vi "Sequencer.vi"() -> ()   [LabVIEW 2019]
uses:
  Sequencer mode.ctl
  Axis driver/Xeryon Axis command.ctl
  Serial driver/Xeryon serial command.ctl
panel:
  in  "Exit":bool
  out "Within tolerance":bool
  in  "Stop":bool
  in  "Apply default file":bool
  in  "Settings default":path
  out "Position reached":bool
  in  "Stage selector":string
  out "Current pos":dbl
  in  "# cycles":u16
  out "Cycle":u16
  in  "Speed":dbl
  in  "Position 2":dbl
  in  "Position 1":dbl
  in  "Start":bool
  in  "Current status":T1
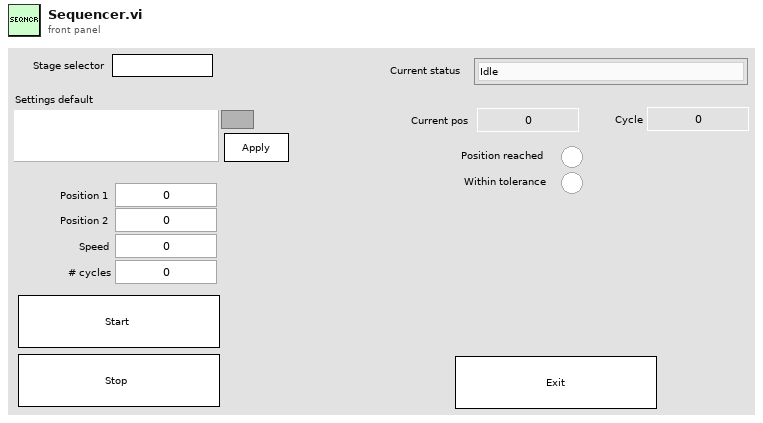
[diagram p1: front panel]
types:
  T1 = typedef "Sequencer mode.ctl" = enum16{"Idle", "-", "Go to first pos", "Moving to first position", "Go to 2nd pos", "Moving to 2nd position", "Check what's next"}
  T2 = typedef "Xeryon Axis command.ctl" = cluster{"Command":enum16{"Reset", "Zero output", "Go home", "Find index", "Scan -X", "Scan +X", "Scan Stop", "Step -X", "Step +X", "Set DPOS", "Stop", "Continue", "Desired speed", "Apply settings file", "Exit", "Reset encoder", "Recover", "Save"}, "Data to send":string}
  T3 = typedef "Xeryon serial command.ctl" = cluster{"Command":enum16{"Send serial data", "Exit"}, "Data to send":string}
  T4 = enum16{"Init", "Set stage data", "Update position", "Get"}
  T5 = typedef "Xeryon status bits.ctl" = cluster{"Amplifiers enabled":bool, "End stop":bool, "Thermal protection 1":bool, "Thermal protection 2":bool, "Force zero":bool, "Motor On":bool, "Closed loop":bool, "Encoder at index":bool, "Encoder valid":bool, "Searching index":bool, "Position reached":bool, "Error compensation":bool, "Encoder error":bool, "Scanning":bool, "Left end stop":bool, "Right and stop":bool, "Error limit":bool, "Searching optimal frequency":bool, "Safety timeout triggered":bool, "EtherCAT acknowledge":bool, "Emergency stop":bool, "Position fail":bool}
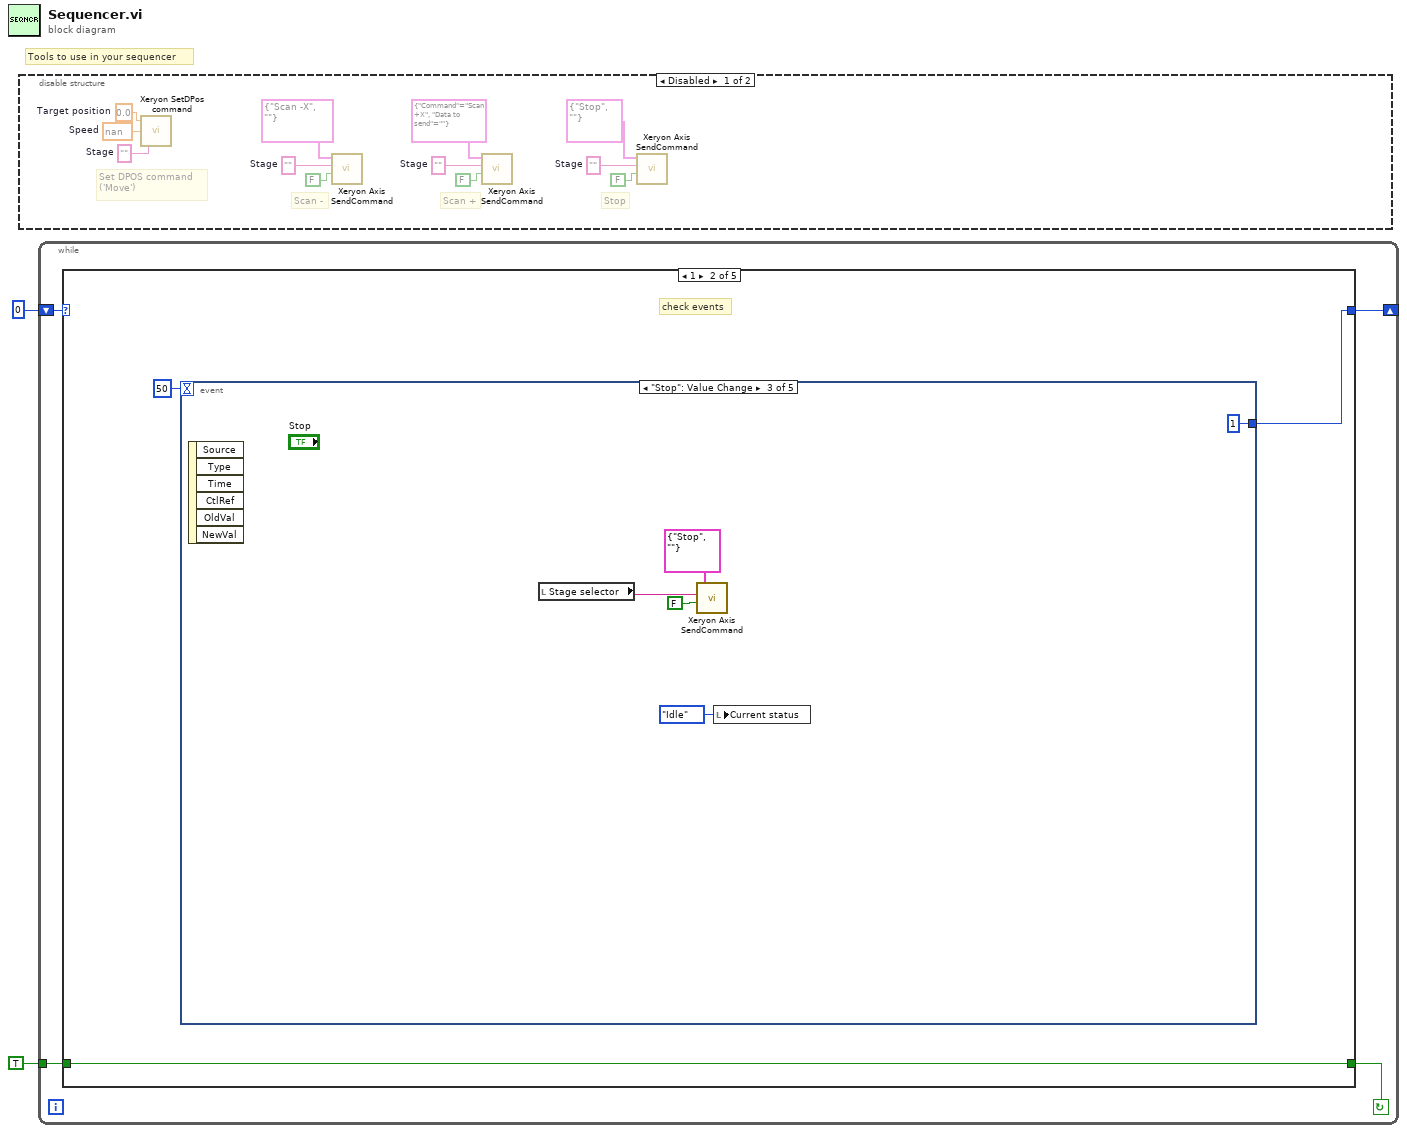
[diagram p0: block diagram]
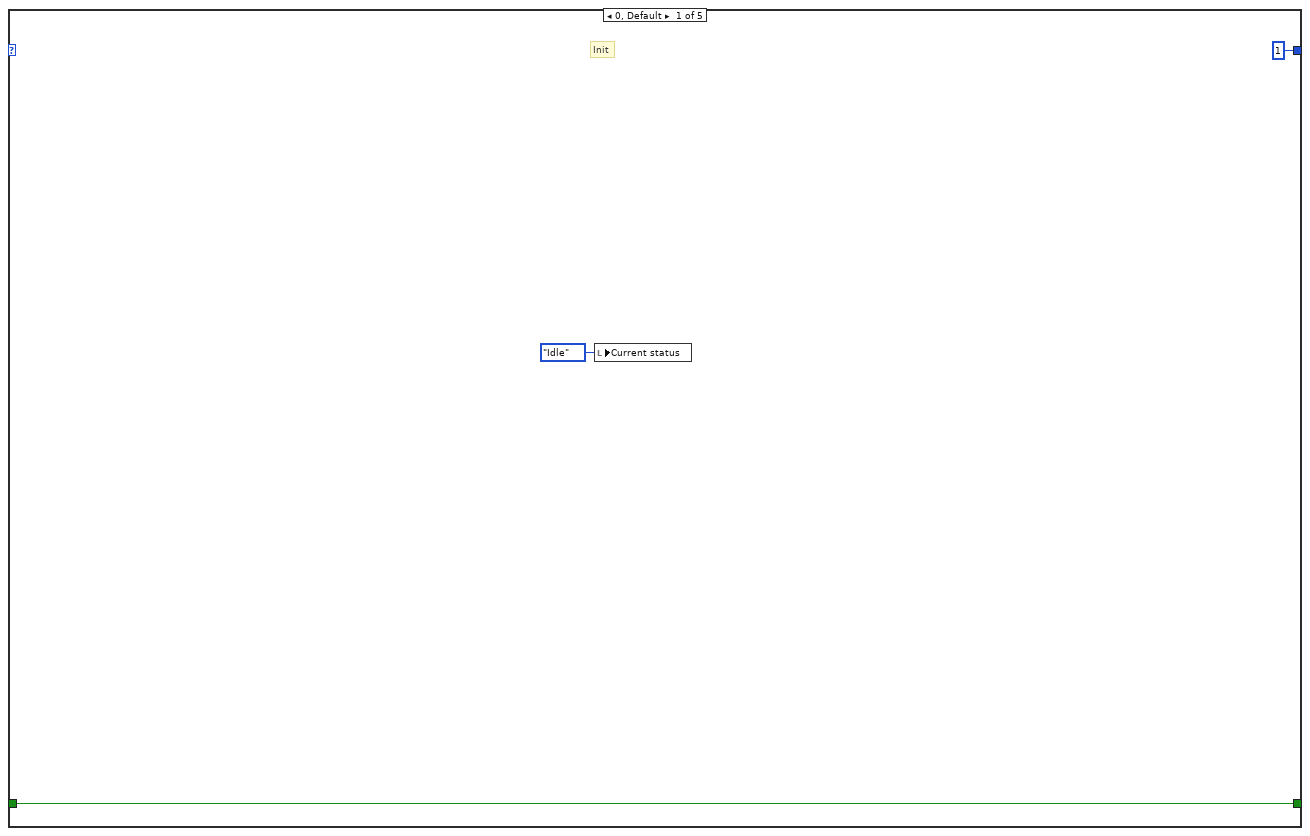
[diagram p3: hidden frame]
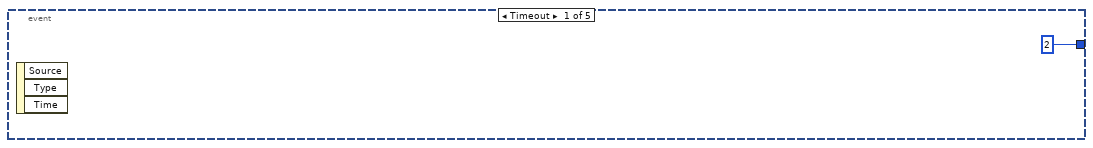
[diagram p4: hidden frame]
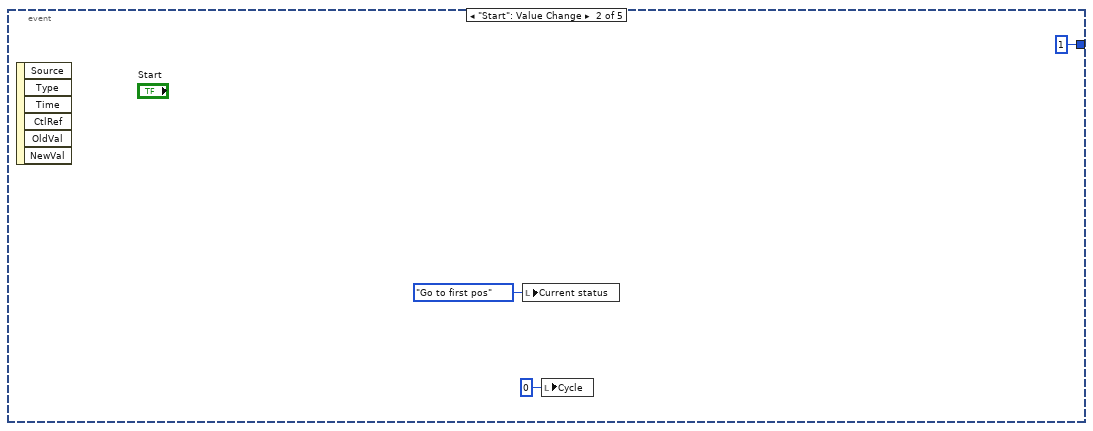
[diagram p5: hidden frame]
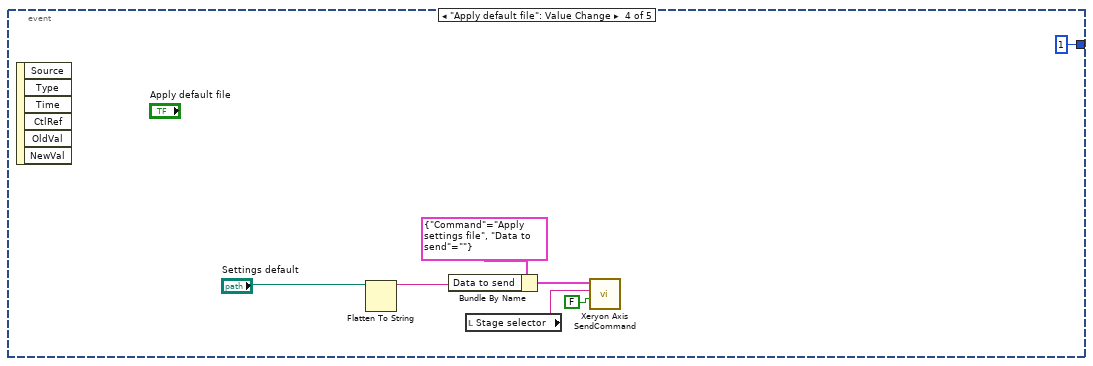
[diagram p6: hidden frame]
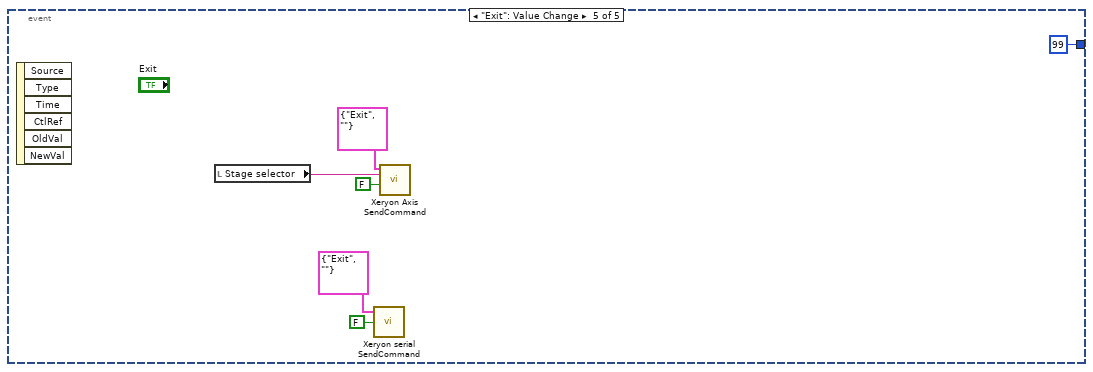
[diagram p7: hidden frame]
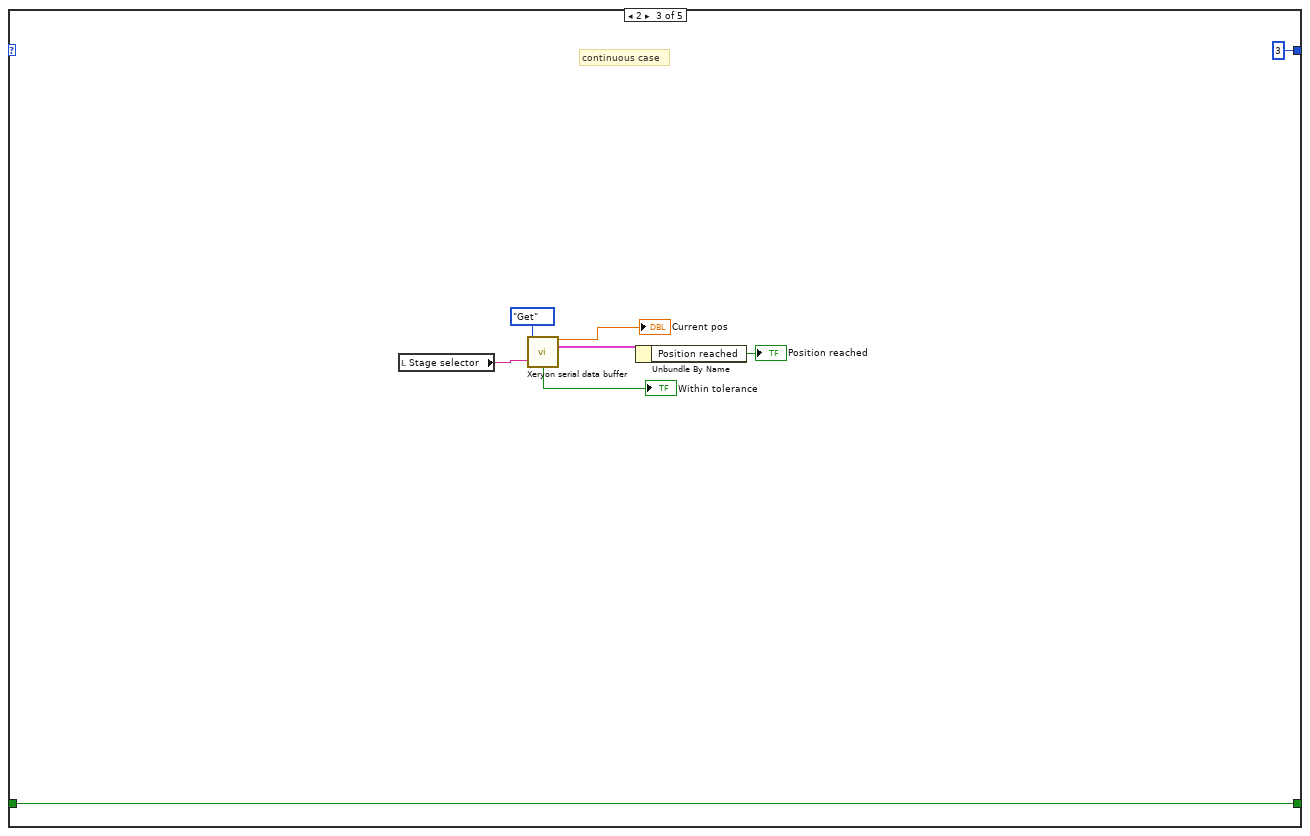
[diagram p8: hidden frame]
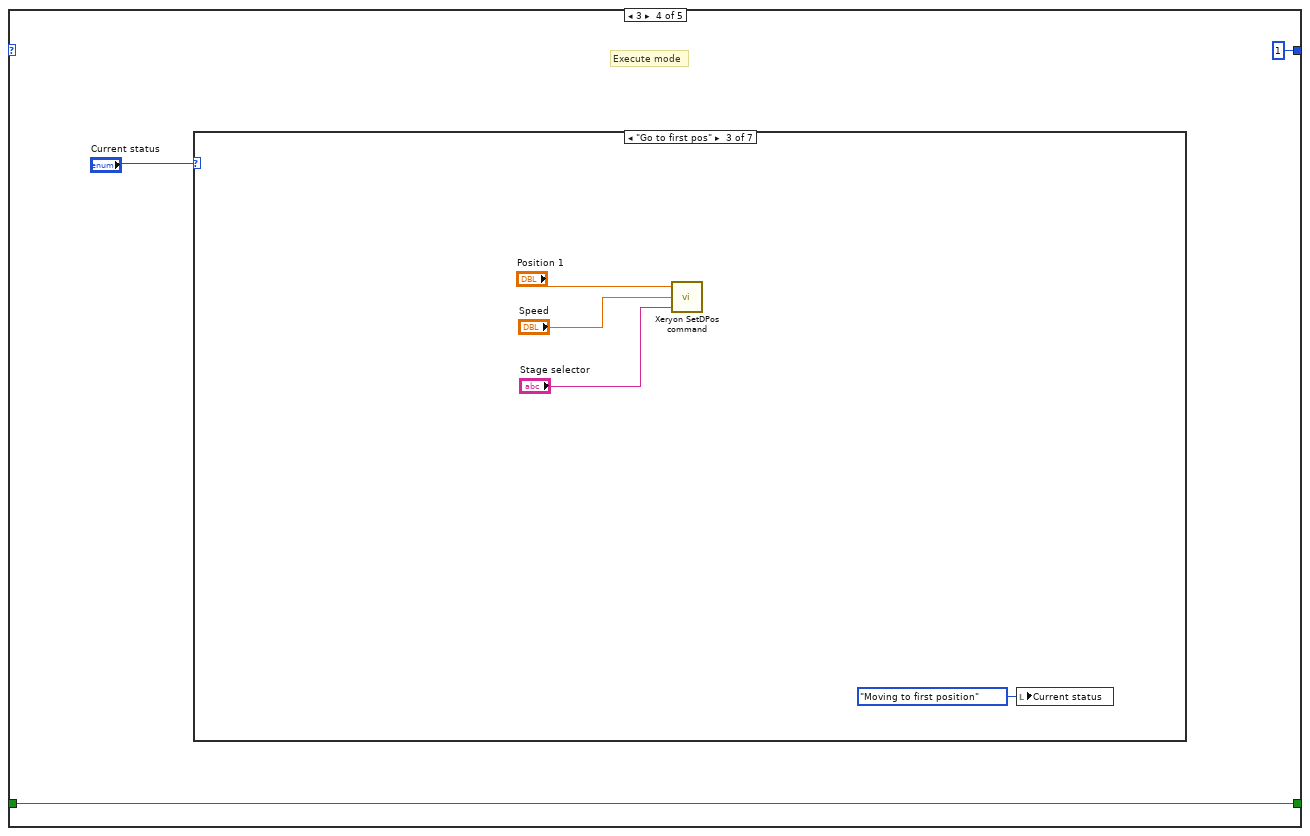
[diagram p9: hidden frame]
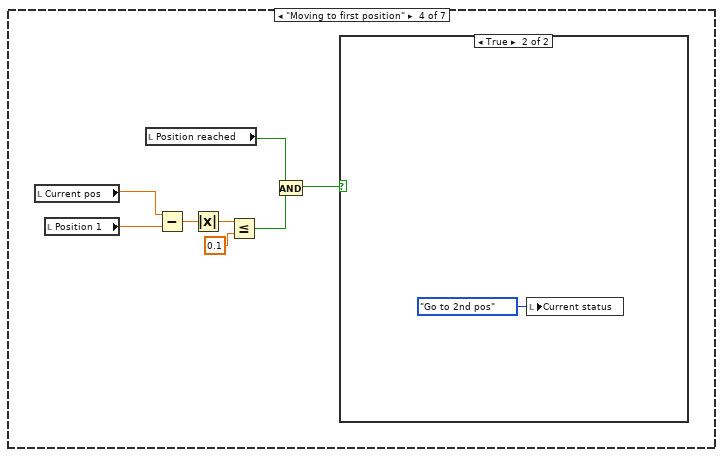
[diagram p12: hidden frame]
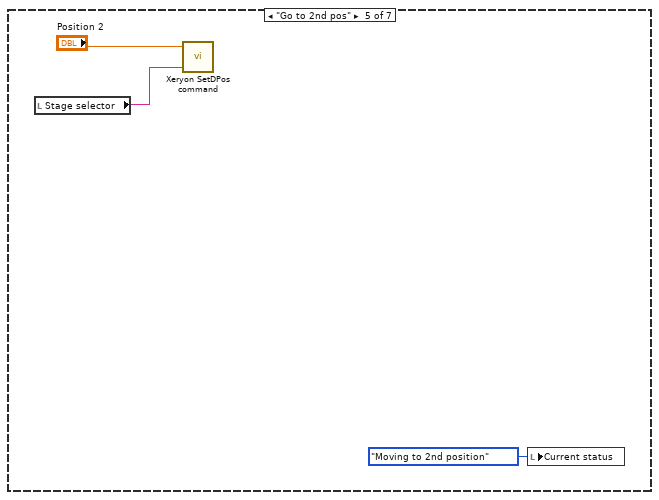
[diagram p14: hidden frame]
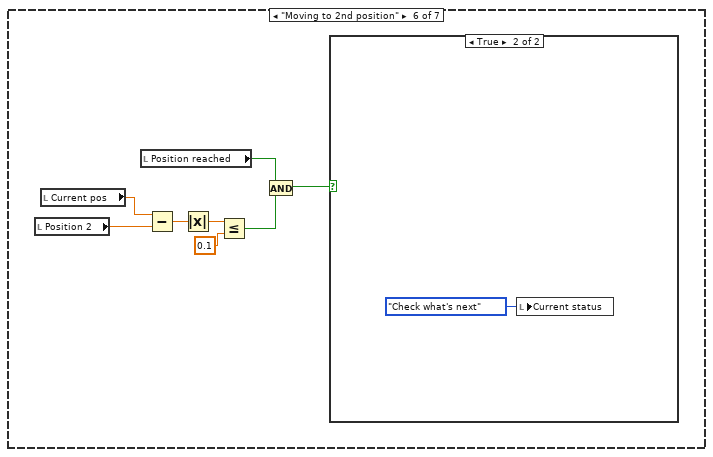
[diagram p15: hidden frame]
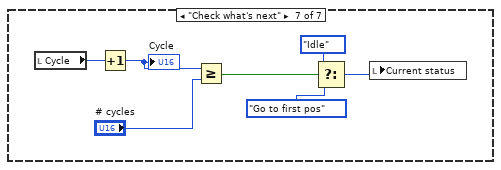
[diagram p17: hidden frame]
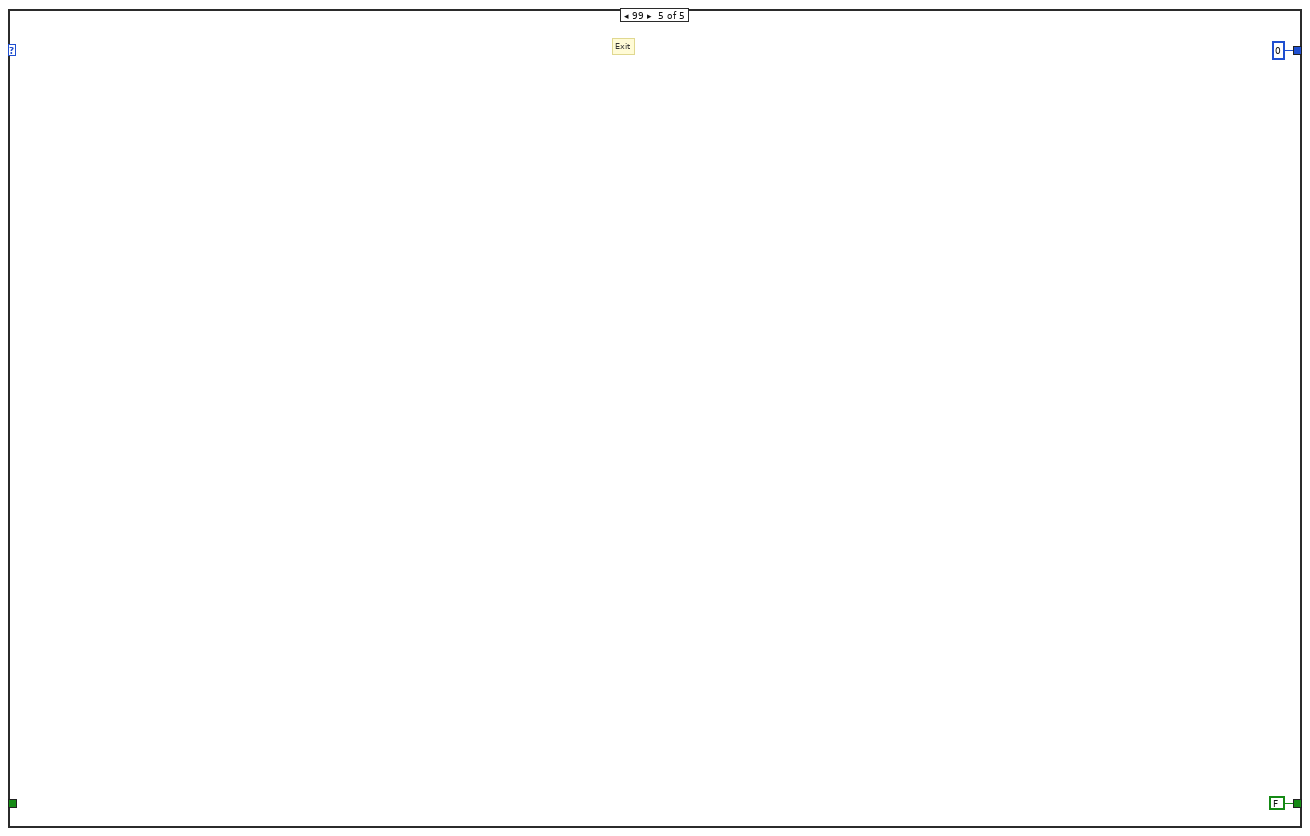
[diagram p18: hidden frame]
diagram:
  # "Tools to use in your sequencer"
  n1 = disable-structure shown="Disabled" {
    frame Disabled {
      w4 = ""  # Stage
      w7 = ""  # Stage
      w9 = ""  # Stage
      w10 = nan  # Speed
      w11 = 0.0  # Target position
      w13 = ""  # Stage
      # "Stop"
      # "Scan +"
      # "Scan -"
      # "Set DPOS command\n('Move')"
      n2 = call "Xeryon SetDPos command.vi"("Stage"=w9, "Speed"=w10, "Target position"=w11) -> ()  [unwired: 3 in]
      n3 = call "Xeryon Axis SendCommand.vi"("Feedback?"=FALSE, "Stage"=w13, "Axis Command"=T2 {"Command"=enum."Scan -X", "Data to send"=""}) -> ()  [unwired: 3 in, 1 out]
      n4 = call "Xeryon Axis SendCommand.vi"("Feedback?"=FALSE, "Stage"=w7, "Axis Command"=T2 {"Command"=enum."Scan +X", "Data to send"=""}) -> ()  [unwired: 3 in, 1 out]
      n5 = call "Xeryon Axis SendCommand.vi"("Feedback?"=FALSE, "Stage"=w4, "Axis Command"=T2 {"Command"=enum."Stop", "Data to send"=""}) -> ()  [unwired: 3 in, 1 out]
    }
    frame Enabled {
    }
  }
  n6 = while {
    shift-right: [w15] -> _
    shift-left: 0 -> [w18]
    tunnel: TRUE -> [w17]
    stop <- w16 continue-if-true
    n7 = case shown="1" w18 {
      tunnel: [w21 w24 w54 w56 FALSE] -> w16
      tunnel: w17 -> [w21 w24 w54 w56 _]
      tunnel: [1 w22 3 1 0] -> w15
      frame 0, Default {
        # "Init"
        n8 = local write "Current status"(Sequencer_mode."Idle" ("Current mode")) -> ()
      }
      frame 1 {
        # "check events"
        n9 = event shown="[2] \"Stop\": Value Change" {
          selector: _ -> [_ _ _ _ _]
          dyn-events: _ -> [_ _ _ _ _]
          timeout: 50 -> [_ _ _ _ _]
          tunnel: [2 1 1 1 99] -> w22
          event Timeout {
            n10 = event-data() -> ()  [unwired: 1 in, 3 out]
          }
          event "Start": Value Change {
            n11 = event-data() -> ()  [unwired: 1 in, 6 out]
            n12 = local write "Current status"(Sequencer_mode."Go to first pos" ("Current status")) -> ()
            n13 = local write "Cycle"(u16 0 ("Cycle")) -> ()
          }
          event "Stop": Value Change {
            n14 = event-data() -> ()  [unwired: 1 in, 6 out]
            n15 = local read "Stage selector"() -> (w30:string)
            n16 = call "Xeryon Axis SendCommand.vi"("Feedback?"=FALSE, "Stage"=w30, "Axis Command"=T2 {"Command"=enum."Stop", "Data to send"=""} ("Axis Message")) -> ()  [unwired: 3 in, 1 out]
            n17 = local write "Current status"(Sequencer_mode."Idle" ("Current status")) -> ()
          }
          event "Apply default file": Value Change {
            n18 = event-data() -> ()  [unwired: 1 in, 6 out]
            n19 = Flatten To String(anything="Settings default") -> (data string=w37:string)  [unwired: 3 in, 2 out]
            n20 = Bundle By Name(cluster=T2 {"Command"=enum."Apply settings file", "Data to send"=""} ("Axis Message"), "Data to send"=w37) -> (w36:T2)
            n21 = local read "Stage selector"() -> (w34:string)
            n22 = call "Xeryon Axis SendCommand.vi"("Feedback?"=FALSE, "Stage"=w34, "Axis Command"=w36) -> ()  [unwired: 3 in, 1 out]
          }
          event "Exit": Value Change {
            n23 = event-data() -> ()  [unwired: 1 in, 6 out]
            n24 = local read "Stage selector"() -> (w41:string)
            n25 = call "Xeryon serial SendCommand.vi"("Feedback?"=FALSE, "Serial Command"=T3 {"Command"=enum."Exit", "Data to send"=""} ("Serial Message")) -> ()  [unwired: 1 in, 3 out]
            n26 = call "Xeryon Axis SendCommand.vi"("Feedback?"=FALSE, "Stage"=w41, "Axis Command"=T2 {"Command"=enum."Exit", "Data to send"=""} ("Axis Message")) -> ()  [unwired: 3 in, 1 out]
          }
        }
      }
      frame 2 {
        # "continuous case"
        n27 = local read "Stage selector"() -> (w52:string)
        n28 = call "Xeryon serial data buffer.vi"("Mode"=T4."Get", "Select drive letter"=w52) -> ("Position out"=→"Current pos":dbl, "Statusbits out"=w49:T5, "Within tol out"=→"Within tolerance":bool)  [unwired: 7 in, 4 out]
        n29 = Unbundle By Name(w49) -> ("Position reached"=→"Position reached":bool)
      }
      frame 3 {
        # "Execute mode"
        n30 = case shown="\"Go to first pos\"" "Current status" {
          frame "Idle", Default {
          }
          frame "-" {
          }
          frame "Go to first pos" {
            n31 = call "Xeryon SetDPos command.vi"("Stage"="Stage selector", "Speed"="Speed", "Target position"="Position 1") -> ()  [unwired: 3 in]
            n32 = local write "Current status"(Sequencer_mode."Moving to first position" ("Current status")) -> ()
          }
          frame "Moving to first position" {
            n33 = local read "Current pos"() -> (w63:dbl)
            n34 = local read "Position 1"() -> (w69:dbl)
            n35 = local read "Position reached"() -> (w62:bool)
            n36 = Subtract(x=w63, y=w69) -> (x-y=w68:dbl)
            n37 = Absolute Value(x=w68) -> (abs(x)=w67:dbl)
            n38 = Less Or Equal?(x=w67, y=0.1) -> (x <= y?=w65:bool)
            n39 = And(x=w62, y=w65) -> (x .and. y?=w64:bool)
            n40 = case shown="True" w64 {
              frame False {
              }
              frame True {
                n41 = local write "Current status"(Sequencer_mode."Go to 2nd pos" ("Current status")) -> ()
              }
            }
          }
          frame "Go to 2nd pos" {
            n42 = local read "Stage selector"() -> (w72:string)
            n43 = call "Xeryon SetDPos command.vi"("Stage"=w72, "Target position"="Position 2") -> ()  [unwired: 4 in]
            n44 = local write "Current status"(Sequencer_mode."Moving to 2nd position" ("Current status")) -> ()
          }
          frame "Moving to 2nd position" {
            n45 = local read "Position 2"() -> (w81:dbl)
            n46 = local read "Current pos"() -> (w75:dbl)
            n47 = local read "Position reached"() -> (w74:bool)
            n48 = Subtract(x=w75, y=w81) -> (x-y=w80:dbl)
            n49 = Absolute Value(x=w80) -> (abs(x)=w79:dbl)
            n50 = Less Or Equal?(x=w79, y=0.1) -> (x <= y?=w77:bool)
            n51 = And(x=w74, y=w77) -> (x .and. y?=w76:bool)
            n52 = case shown="True" w76 {
              frame False {
              }
              frame True {
                n53 = local write "Current status"(Sequencer_mode."Check what's next" ("Current status")) -> ()
              }
            }
          }
          frame "Check what's next" {
            n54 = local read "Cycle"() -> (w89:u16)
            n55 = Increment(x=w89) -> (x+1=w88:u16)
            "Cycle" <- w88
            n56 = Greater Or Equal?(x=w88, y="# cycles") -> (x >= y?=w86:bool)
            n57 = Select(t=Sequencer_mode."Idle" ("Current status"), s=w86, f=Sequencer_mode."Go to first pos" ("Current status")) -> (s? t:f=w83:T1)
            n58 = local write "Current status"(w83) -> ()
          }
        }
      }
      frame 99 {
        # "Exit"
      }
    }
  }
